vi "Slide-Motor_Api.vi"(8 "Error In":errorcluster, 11 "移動距離":dbl=35.0) -> (0 "Error Out":errorcluster)   [LabVIEW 2019]
uses:
  <vilib>/Platform/TimedLoop/XDataNode/timing_clust.ctl
  <vilib>/Platform/TimedLoop/XDataNode/nitl_modes.ctl
  <vilib>/Platform/TimedLoop/XDataNode/wakeup.ctl
  Variable/Lock-PID.vi
  <vilib>/platform/TimedLoop/XDataNode/XDataNode.xnode
  <vilib>/Platform/TimedLoop/XDataNode/XDNodeRunTimeDep.lvlib
panel:
  out "Waveform Chart":dbl(graph)
  out "移動角度":dbl
  in  "Stop":bool
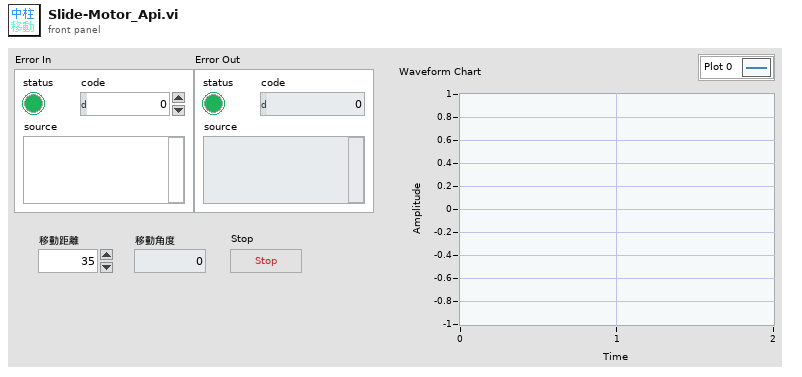
[diagram p1: front panel]
types:
  T1 = typedef "XDNodeRunTimeDep.lvlib/timing_clust.ctl" = cluster{"Expected End [f-1]":u64, "Actual End [f-1]":u64, "Finished Late? [f-1]":bool, "Expected End [i-1]":u64, "Actual End [i-1]":u64, "Finished Late? [i-1]":bool, "Expected Start [i]":u64, "Actual Start [i]":u64, "Expected Start [f]":u64, "Actual Start [f]":u64, "Source Name":string, "Structure Name":string, "Period":i64, "Deadline":i64, "Offset":i64, "Start":i64, "Priority":i32, "Timeout":i32, "Mode":T2, "Wakeup Reason":T3, "Error":errorcluster, "Source Type":string, "Secondary Source Type":string, "Global End Time":u64, "Global Start Time":u64, "Frame Duration":u64, "Iteration Duration":u64, "Assigned CPU":i32, "I/O Scan Engine Mode":u32}
  T2 = typedef "XDNodeRunTimeDep.lvlib/nitl_modes.ctl" = enum32{"No Change", "Process missed periods, maintain original phase", "Discard missed periods, maintain original phase", "Process missed periods, ignore original phase", "Discard missed periods, ignore original phase"}
  T3 = typedef "XDNodeRunTimeDep.lvlib/wakeup.ctl" = enum32{"Normal", "Aborted", "Asynchronous wakeup", "Timing source error", "Timed loop error", "Timeout"}
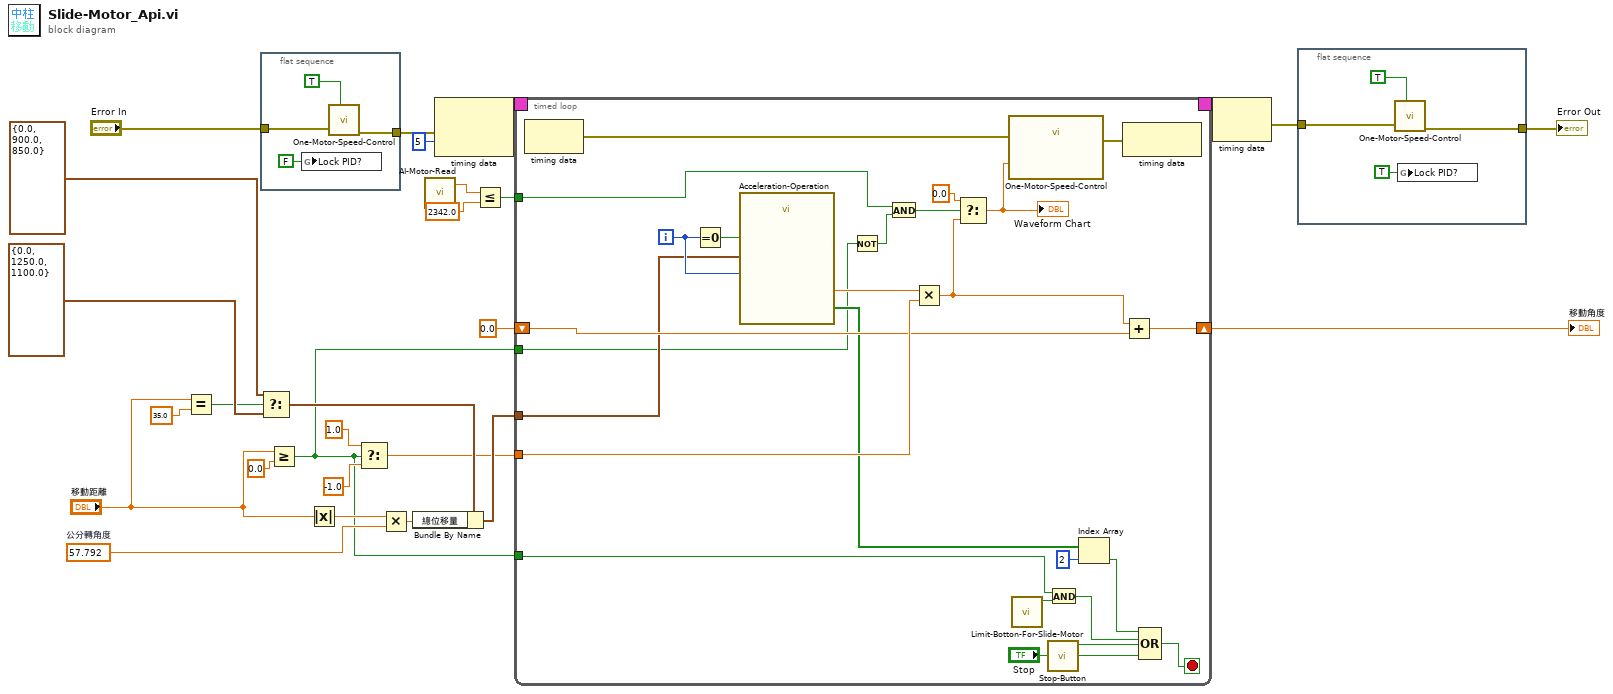
[diagram p0: block diagram]
diagram:
  w7 = 57.792  # 公分轉角度
  n1 = Equal?(x="移動距離", y=35.0) -> (x = y?=w19:bool)
  n2 = flat-sequence {
    tunnel: "Error In" -> [w30]
    tunnel: [w29] -> w11
    frame #0 {
      n3 = global write "Lock-PID.vi" "Lock PID?"(FALSE ("Lock PID?")) -> ()
      n4 = call "One-Motor-Speed-Control.vi"("Reset"=TRUE, "Error In"=w30) -> ("Error Out"=w29:errorcluster)  [unwired: 9 in]
    }
  }
  n5 = Select(t=cluster{"總位移量":dbl, "最高速":dbl, "加速度":dbl} {"總位移量"=0.0, "最高速"=900.0, "加速度"=850.0} ("計算設置"), s=w19, f=cluster{"總位移量":dbl, "最高速":dbl, "加速度":dbl} {"總位移量"=0.0, "最高速"=1250.0, "加速度"=1100.0} ("計算設置")) -> (s? t:f=w21:cluster{"總位移量":dbl, "最高速":dbl, "加速度":dbl})
  n6 = Greater Or Equal?(x="移動距離", y=0.0) -> (x >= y?=w4:bool)
  n7 = Absolute Value(x="移動距離") -> (abs(x)=w13:dbl)
  n8 = Select(t=1.0, s=w4, f=-1.0) -> (s? t:f=w15:dbl)
  n9 = Multiply(x=w13, y=w7) -> (x*y=w14:dbl)
  n10 = Bundle By Name(cluster=w21, "總位移量"=w14) -> (w20:cluster{"總位移量":dbl, "最高速":dbl, "加速度":dbl})
  n11 = call "AI-Motor-Read.vi"() -> ("Data"=w2:dbl)  [unwired: 10 in, 1 out]
  n12 = node-c288(w11, i64 5 ("Period")) -> (w27:T1)
  n13 = Less Or Equal?(x=w2, y=2342.0) -> (x <= y?=w1:bool)
  n14 = timed-loop {
    timing: w27 -> [_]
    timing-out: [_] -> w26
    tunnel: w20 -> [w41]
    tunnel: w15 -> [w49]
    shift-right: [w48] -> w5
    shift-left: 0.0 -> [w47]
    tunnel: w4 -> [w45]
    tunnel: w4 -> [w35]
    tunnel: w1 -> [w34]
    i -> [w42]
    stop <- w56 stop-if-true
    n15 = node-c288() -> (w54:errorcluster)  [unwired: 1 in]
    n16 = Equal To 0?(x=w42) -> (x = 0?=w40:bool)
    n17 = call "Acceleration-Operation.vi"("Reset"=w40, "迴圈( I )"=w42, "計算設置"=w41) -> ("完成?"=w44:bool[], "速度"=w43:dbl)  [unwired: 6 in, 1 out]
    n18 = Not(x=w35) -> (.not. x?=w36:bool)
    n19 = And(x=w34, y=w36) -> (x .and. y?=w37:bool)
    n20 = Multiply(x=w43, y=w49) -> (x*y=w33:dbl)
    n21 = Select(t=0.0, s=w37, f=w33) -> (s? t:f=w32:dbl)
    "Waveform Chart" <- w32
    n22 = call "One-Motor-Speed-Control.vi"("Error In"=w54, "速度(秒/度)"=w32) -> ("Error Out"=w53:errorcluster)  [unwired: 9 in]
    n23 = call "Limit-Botton-For-Slide-Motor.vi"() -> ("中柱微動觸發?"=w39:bool)  [unwired: 10 in, 1 out]
    n24 = call "Stop-Button.vi"() -> ("顯示按下?"=w55:bool)  [unwired: 10 in, 1 out]
    n25 = And(x=w45, y=w39) -> (x .and. y?=w46:bool)
    n26 = Index Array(array=w44, index=2) -> (element=w51:bool)
    n27 = node-c288(w53) -> ()  [unwired: 1 out]
    n28 = Add(x=w33, y=w47) -> (x+y=w48:dbl)
    n29 = Compound Arithmetic op=OR(w51, w46, w55, "Stop") -> (w56:bool)
  }
  "移動角度" <- w5
  n30 = node-c288(w26) -> (w10:errorcluster)
  n31 = flat-sequence {
    tunnel: w10 -> [w64]
    tunnel: [w63] -> w9
    frame #0 {
      n32 = call "One-Motor-Speed-Control.vi"("Reset"=TRUE, "Error In"=w64) -> ("Error Out"=w63:errorcluster)  [unwired: 9 in]
      n33 = global write "Lock-PID.vi" "Lock PID?"(TRUE ("Lock PID?")) -> ()
    }
  }
  "Error Out" <- w9
